vi "1port_Save Parametric Data to csv.vi"(0 "Filepath":path=path "C:/Users/Eddie.Rickey/Desktop/Test Data", 1 "Date Cluster":T6, 3 "PreTest Capacitance":dbl[](array[numeric]), 5 "Test Information":T7={"Exp Name"="Cold Switching", "Lot"="0233A", "Wafer"="15", "Die Type"="L22", "Die X "="6", "Die Y"="8", "Exp"="1", "Die X_Y"="8"}, 7 "Specific Voltages":dbl[](array[numeric])=[32.0, 36.0], 9 "Parametric Calculated Values":T1, 11 "error in (no error)":errorcluster, 12 "Meas Type":string, 14 "PostTest Capacitance":dbl[](array[numeric])) -> (15 "error out":errorcluster)   [LabVIEW 2013]
uses:
  Controls/Test Information.ctl
  Controls/Date Control.ctl
  Controls/1 port_Parametric Calculated Values.ctl
  Controls/Port Capacitance Parametric Calculations.ctl
  Controls/Port Voltage Parametric Calculations.ctl
  Controls/Port Resistance Parametric Calculations.ctl
  Controls/Resistance Array Calculated Values.ctl
  <vilib>/Utility/file.llb/Write To Spreadsheet File (string).vi
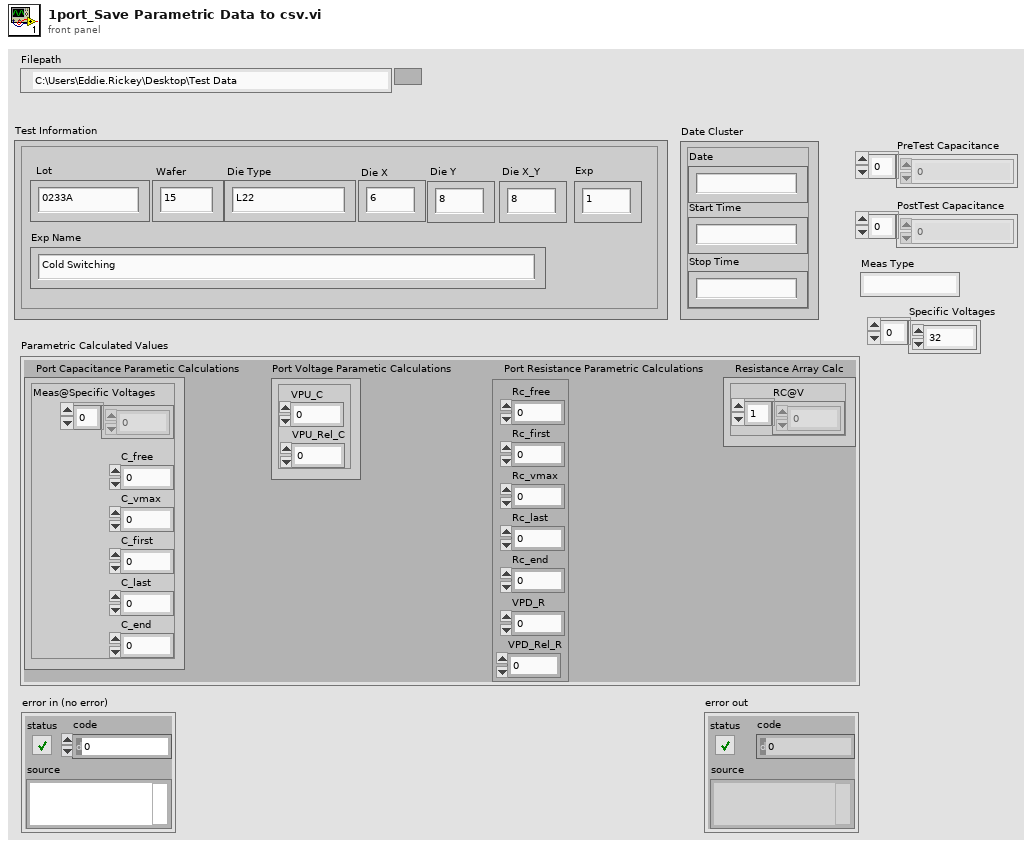
[diagram p1: front panel]
types:
  T1 = typedef "1 port_Parametric Calculated Values.ctl" = cluster{"Port Capacitance Parametic Calculations":T2, "Port Voltage Parametic Calculations":T3, "Port Resistance Parametric Calculations":T4, "Resistance Array Calc":T5}
  T2 = typedef "Port Capacitance Parametric Calculations.ctl" = cluster{"C_free":dbl, "C_vmax":dbl, "C_first":dbl, "C_last":dbl, "C_end":dbl, "Meas@Specific Voltages":dbl[]}
  T3 = typedef "Port Voltage Parametric Calculations.ctl" = cluster{"VPU_C":dbl, "VPU_Rel_C":dbl}
  T4 = typedef "Port Resistance Parametric Calculations.ctl" = cluster{"Rc_free":dbl, "Rc_first":dbl, "Rc_vmax":dbl, "Rc_last":dbl, "Rc_end":dbl, "VPD_R":dbl, "VPD_Rel_R":dbl}
  T5 = typedef "Resistance Array Calculated Values.ctl" = cluster{"RC@V":dbl[]}
  T6 = typedef "Date Control.ctl" = cluster{"Date":string, "Start Time":string, "Stop Time":string}
  T7 = typedef "Test Information.ctl" = cluster{"Exp Name":string, "Lot":string, "Wafer":string, "Die Type":string, "Die X ":string, "Die Y":string, "Exp":string, "Die X_Y":string}
  T8 = enum16{"open", "replace", "create", "open or create", "replace or create", "replace or create with confirmation"}
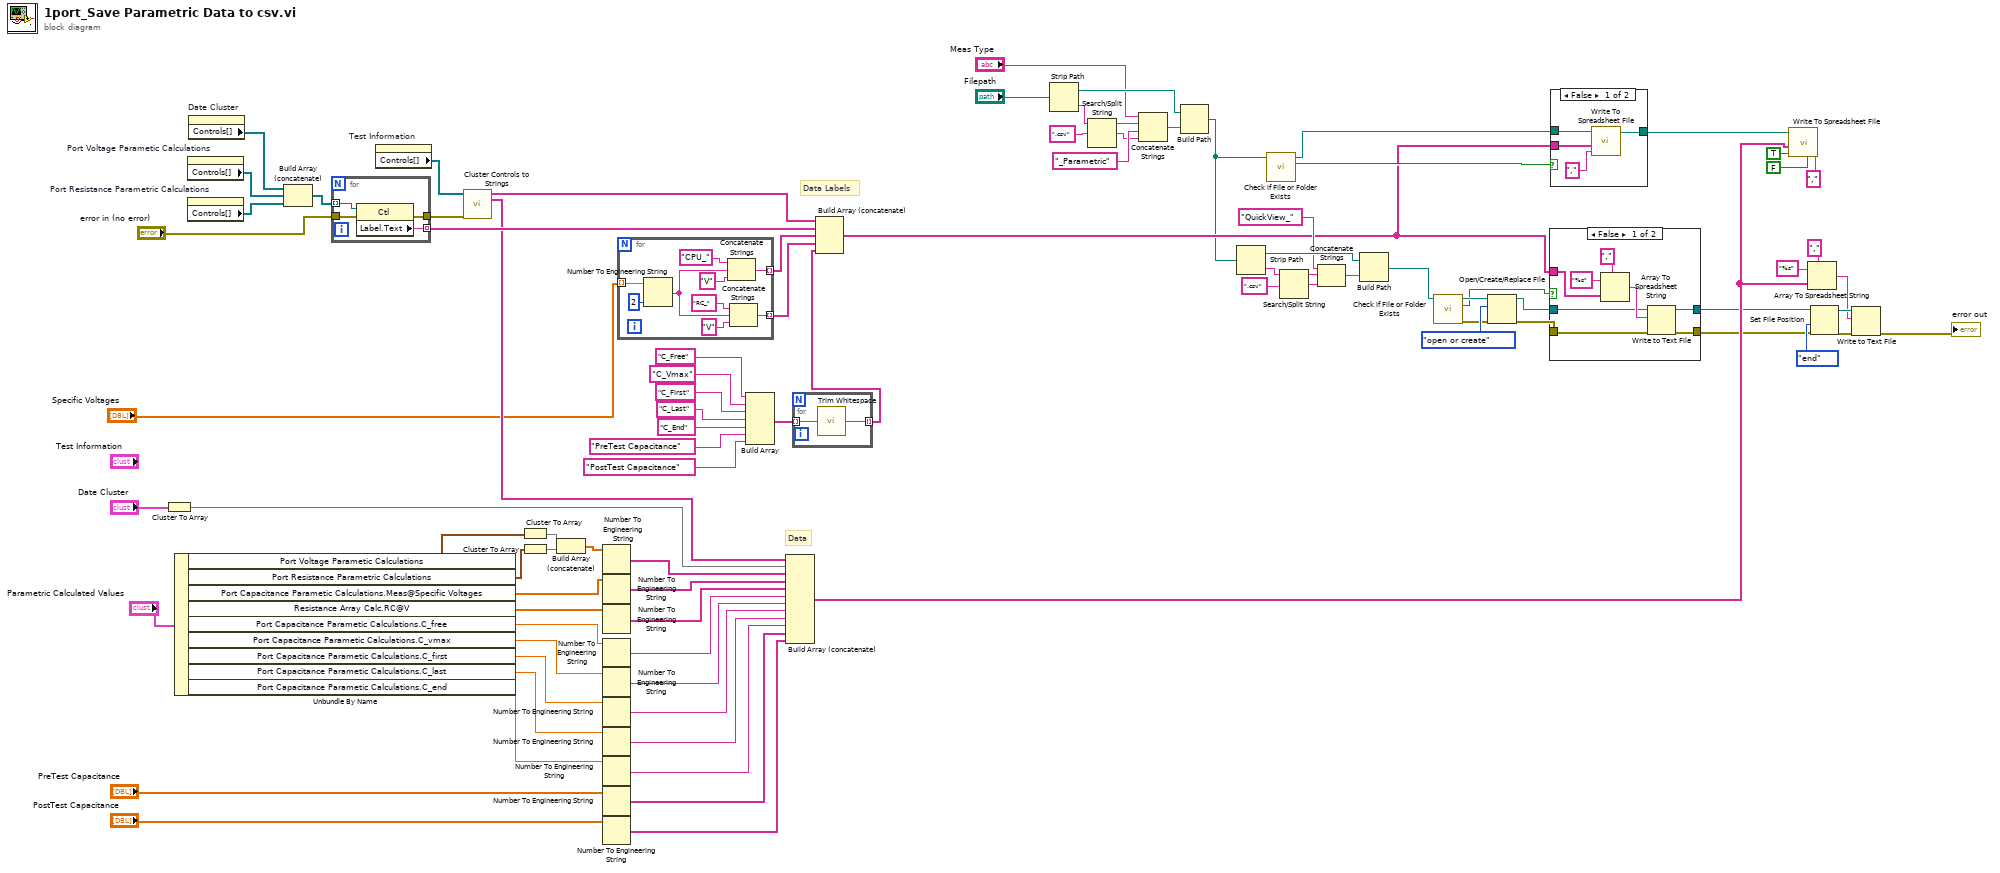
[diagram p0: block diagram]
diagram:
  # "Data"
  # "Data Labels"
  n1 = Cluster To Array(cluster="Date Cluster") -> (array=w67:string[])
  n2 = Unbundle By Name("Parametric Calculated Values") -> ("Port Voltage Parametic Calculations"=w34:T3, "Port Resistance Parametric Calculations"=w33:T4, "Port Capacitance Parametic Calculations.Meas@Specific Voltages"=w9:dbl[], "Resistance Array Calc.RC@V"=w7:dbl[], "Port Capacitance Parametic Calculations.C_free"=w32:dbl, "Port Capacitance Parametic Calculations.C_vmax"=w28:dbl, "Port Capacitance Parametic Calculations.C_first"=w27:dbl, "Port Capacitance Parametic Calculations.C_last"=w26:dbl, "Port Capacitance Parametic Calculations.C_end"=w25:dbl)
  n3 = property on="Port Voltage Parametic Calculations" class="Clust (strict)"() -> ("Controls[]"=w31:refnum<vi>[])  [unwired: 2 in, 2 out]
  n4 = property on="Port Resistance Parametric Calculations" class="Clust (strict)"() -> ("Controls[]"=w30:refnum<vi>[])  [unwired: 2 in, 2 out]
  n5 = property on="Date Cluster" class="Clust (strict)"() -> ("Controls[]"=w70:refnum<vi>[])  [unwired: 2 in, 2 out]
  n6 = Build Array (concatenate)(w70, w31, w30) -> (w90:refnum<vi>[])
  n7 = for {
    tunnel: [w94] -> w87 mode=indexing
    tunnel: w90 -> [w93] mode=indexing
    tunnel: [w92] -> w86
    tunnel: "error in (no error)" -> [w91]
    n8 = property class="Ctl"(reference=w93, error in=w91) -> (error out=w92:errorcluster, "Label.Text"=w94:string)  [unwired: 1 out]
  }
  n9 = property on="Test Information" class="Clust (strict)"() -> ("Controls[]"=w89:refnum<vi>[])  [unwired: 2 in, 2 out]
  n10 = call "Cluster Controls to Strings.vi"("Controls[]"=w89, "Error In"=w86) -> ("Control Labels"=w88:string[], "Control Values"=w69:string[])  [unwired: 11 in, 1 out]
  n11 = Cluster To Array(cluster=w34) -> (array=w85:dbl[])
  n12 = Cluster To Array(cluster=w33) -> (array=w84:dbl[])
  n13 = Build Array (concatenate)(w85, w84) -> (w83:dbl[])
  n14 = Number To Engineering String(4:w83) -> (0:w10:string[])  [unwired: 3 in]
  n15 = Number To Engineering String(4:w9) -> (0:w8:string[])  [unwired: 3 in]
  n16 = Number To Engineering String(4:w7) -> (0:w6:string[])  [unwired: 3 in]
  n17 = Number To Engineering String(4:w32) -> (0:w82:string)  [unwired: 3 in]
  n18 = Number To Engineering String(4:w28) -> (0:w72:string)  [unwired: 3 in]
  n19 = Number To Engineering String(4:w27) -> (0:w71:string)  [unwired: 3 in]
  n20 = Number To Engineering String(4:w26) -> (0:w23:string)  [unwired: 3 in]
  n21 = Number To Engineering String(4:w25) -> (0:w22:string)  [unwired: 3 in]
  n22 = Number To Engineering String(4:"PreTest Capacitance") -> (0:w21:string[])  [unwired: 3 in]
  n23 = Number To Engineering String(4:"PostTest Capacitance") -> (0:w20:string[])  [unwired: 3 in]
  n24 = for {
    tunnel: "Specific Voltages" -> [w103] mode=indexing
    tunnel: [w96] -> w74 mode=indexing
    tunnel: [w99] -> w73 mode=indexing
    n25 = Number To Engineering String(2:i16 2 ("precision (6)"), 4:w103) -> (0:w97:string)  [unwired: 2 in]
    n26 = Concatenate Strings("CPU_" ("search string"), w97, "V" ("string")) -> (w96:string)
    n27 = Concatenate Strings("RC_" ("search string"), w97, "V" ("string")) -> (w99:string)
  }
  n28 = Build Array("C_Free", "C_Vmax", "C_First", "C_Last", "C_End", "PreTest Capacitance", "PostTest Capacitance") -> (w5:string[])
  n29 = Build Array (concatenate)(w69, w67, w10, w8, w6, w82, w72, w71, w23, w22, w21, w20) -> (w43:string[])
  n30 = for {
    tunnel: w5 -> [w105] mode=indexing
    tunnel: [w104] -> w4 mode=indexing
    n31 = call <vilib>:"Trim Whitespace.vi"("string"=w105) -> ("trimmed string"=w104:string)  [unwired: 1 in]
  }
  n32 = Build Array (concatenate)(w88, w87, w74, w73, w4) -> (w46:string[])
  n33 = Strip Path(path="Filepath") -> (stripped path=w76:path, name=w81:string)
  n34 = Search/Split String(string=w81, search string/char (-)=".csv" ("search string")) -> (substring before match=w79:string, match + rest of string=w77:string)  [unwired: 1 in, 1 out]
  n35 = Concatenate Strings("Meas Type", w79, "_Parametric" ("search string"), w77) -> (w75:string)
  n36 = Build Path(base path=w76, name or relative path=w75) -> (appended path=w2:path)
  n37 = Strip Path(path=w2) -> (stripped path=w62:path, name=w65:string)
  n38 = call <vilib>:"Check if File or Folder Exists.vi"("path"=w2) -> ("file or folder exists?"=w47:bool, "dup path"=w52:path)  [unwired: 8 in, 1 out]
  n39 = Search/Split String(string=w65, search string/char (-)=".csv" ("search string")) -> (substring before match=w60:string, match + rest of string=w63:string)  [unwired: 1 in, 1 out]
  n40 = Concatenate Strings("QuickView_" ("search string"), w60, w63) -> (w61:string)
  n41 = Build Path(base path=w62, name or relative path=w61) -> (appended path=w13:path)
  n42 = call <vilib>:"Check if File or Folder Exists.vi"("path"=w13) -> ("error out"=w16:errorcluster, "file or folder exists?"=w14:bool, "dup path"=w15:path)  [unwired: 8 in]
  n43 = Open/Create/Replace File(file path (use dialog)=w15, error in=w16, operation (0:open)=T8."open or create") -> (refnum out=w44:refnum<file>, error out=w45:errorcluster)  [unwired: 3 in, 1 out]
  n44 = case shown="False" w14 {
    tunnel: w46 -> [w111 _]
    tunnel: w44 -> [w109 w115]
    tunnel: w45 -> [w108 w114]
    tunnel: [w107 w114] -> w42
    tunnel: [w106 w115] -> w41
    frame False {
      n45 = Array To Spreadsheet String(delimiter (Tab)="," ("delimiter (\\t)"), array=w111, 3:"%s" ("format string")) -> (spreadsheet string=w110:string)
      n46 = Write to Text File(file (use dialog)=w109, text=w110, error in=w108) -> (refnum out=w106:refnum<file>, error out=w107:errorcluster)  [unwired: 1 in, 1 out]
    }
    frame True {
    }
  }
  n47 = case shown="False" w47 {
    tunnel: w52 -> [w119 w120]
    tunnel: w46 -> [w118 _]
    tunnel: [w116 w120] -> w48
    frame False {
      n48 = call-poly <vilib>:"Write To Spreadsheet File.vi"("delimiter (\\t)"="," ("delimiter (\\t)"), "1D data"=w118, "file path (dialog if empty)"=w119) -> ("new file path (Not A Path if cancelled)"=w116:path)  [unwired: 5 in]
    }
    frame True {
    }
  }
  n49 = call-poly <vilib>:"Write To Spreadsheet File.vi"("delimiter (\\t)"="," ("delimiter (\\t)"), "transpose? (no:F)"=FALSE, "append to file? (new file:F)"=TRUE, "1D data"=w43, "file path (dialog if empty)"=w48) -> ()  [unwired: 3 in, 1 out]
  n50 = Array To Spreadsheet String(delimiter (Tab)="," ("delimiter (\\t)"), array=w43, 3:"%s" ("format string")) -> (spreadsheet string=w53:string)
  n51 = Set File Position(refnum=w41, from (0:start)=enum16{"start", "end", "current"}."end", error in=w42) -> (refnum out=w54:refnum<file>, error out=w55:errorcluster)  [unwired: 1 in]
  n52 = Write to Text File(file (use dialog)=w54, text=w53, error in=w55) -> (error out=→"error out":errorcluster)  [unwired: 1 in, 2 out]
